vi "axex_save_file.vi"(7 "force operation (ignore error in) (True)":bool=TRUE, 8 "error in":errorcluster, 9 "file overwrite prompt (True)":bool=TRUE, 10 "file path (no path)":path, 11 "AX Excel instance in":T1) -> (0 "error out":errorcluster, 3 "AX Excel instance out":T1)   [LabVIEW 2020, in "AX Excel.lvlib"]
doc: "Call this to save unsaved changes in given file.\nIf current workbook is new workbook (not loaded from file) the file path must be entered.\nIf you want to change the save path from implicit (the path from which it was opened), you can enter new path."
uses:
  AX Excel.lvlib
  axex_instance.ctl
  <vilib>/Utility/error.llb/Error Cluster From Error Code.vi
  <vilib>/ErrorRing/Error Ring.xnode
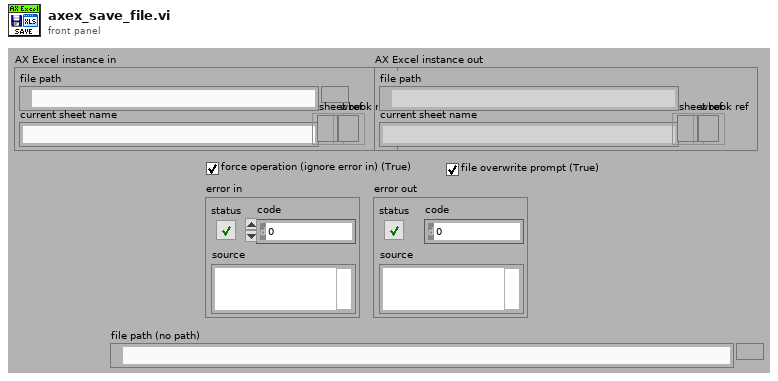
[diagram p1: front panel]
types:
  T1 = typedef "AX Excel.lvlib/axex_instance.ctl" = cluster{"file path":path, "current sheet name":string, "sheet ref":refnum<k7>, "wbook ref":refnum<k7>}
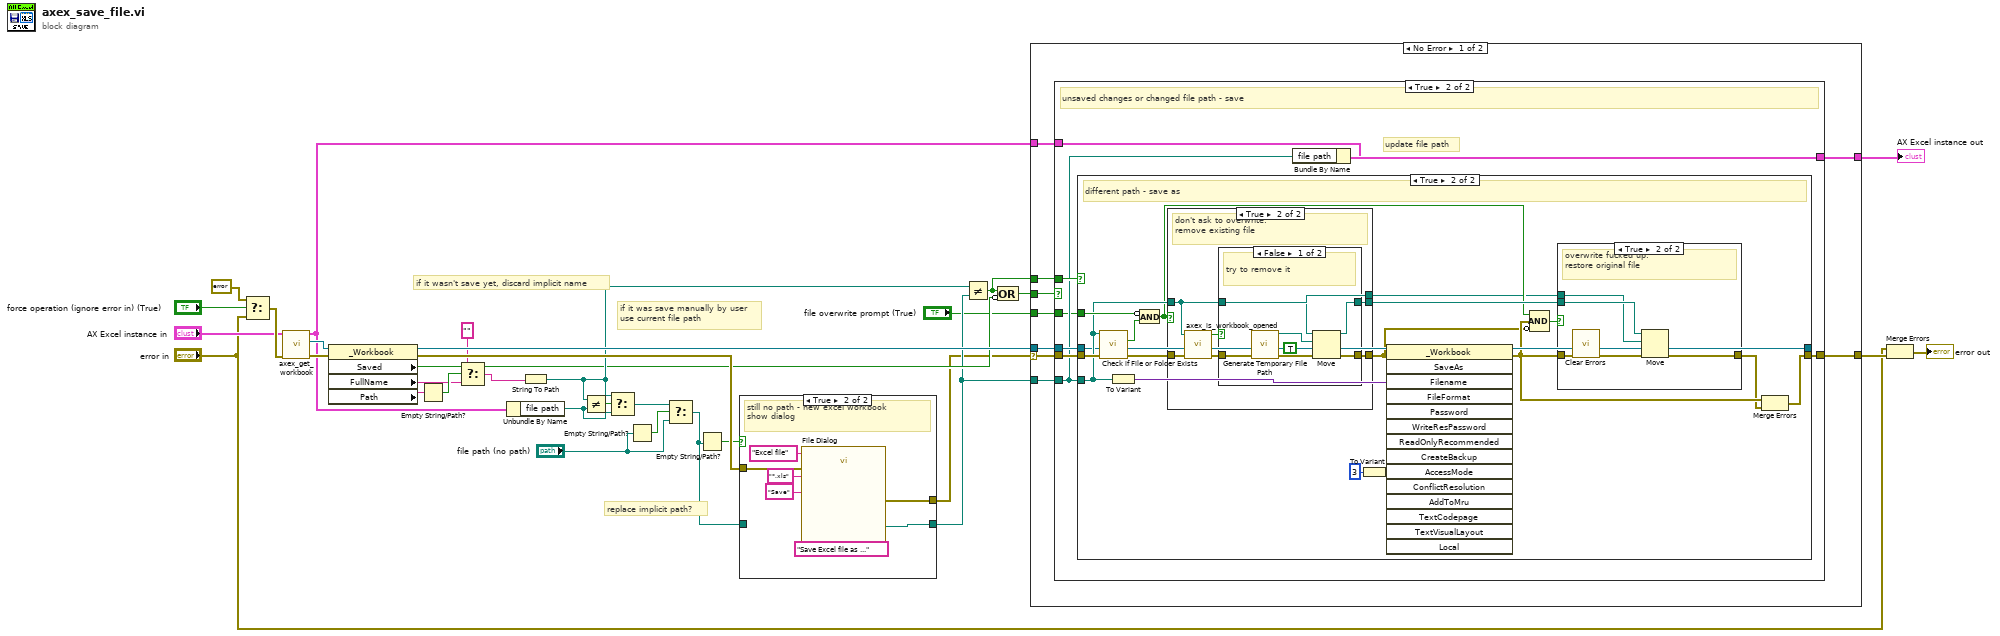
[diagram p0: block diagram]
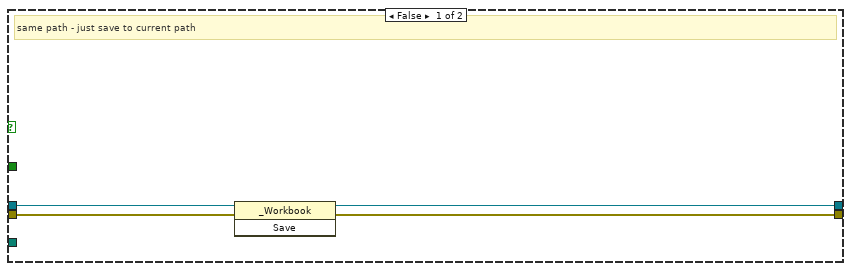
[diagram p3: hidden frame]
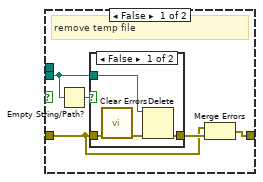
[diagram p4: hidden frame]
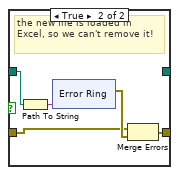
[diagram p7: hidden frame]
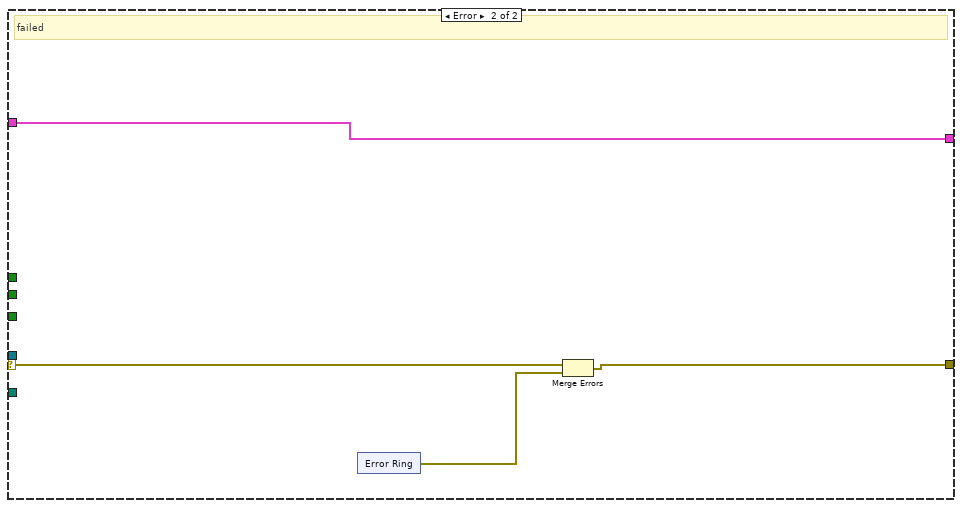
[diagram p8: hidden frame]
diagram:
  # "if it was save manually by user\nuse current file path"
  # "if it wasn't save yet, discard implicit name"
  # "replace implicit path?"
  n1 = Select(t=errorcluster {"status"=FALSE, "code"=0, "source"=""}, s="force operation (ignore error in) (True)", f="error in") -> (s? t:f=w30:errorcluster)
  n2 = call "axex_get_workbook.vi"("error in"=w30, "AX Excel instance in"="AX Excel instance in") -> ("error out"=w32:errorcluster, "excel workbook"=w25:refnum<k7>, "AX Excel instance out"=w8:T1)  [unwired: 7 in]
  n3 = property class="_Workbook"(reference=w25, error in=w32) -> (reference out=w31:refnum<k7>, error out=w19:errorcluster, "Saved"=w14:bool, "FullName"=w4:string, "Path"=w6:string)
  n4 = Empty String/Path?(string/path=w6) -> (empty?=w5:bool)
  n5 = Select(t="", s=w5, f=w4) -> (s? t:f=w2:string)
  n6 = Unbundle By Name(w8) -> ("file path"=w21:path)
  n7 = String To Path(string=w2) -> (path=w15:path)
  n8 = Not Equal?(x=w15, y=w21) -> (x != y?=w22:bool)
  n9 = Select(t=w15, s=w22, f=w21) -> (s? t:f=w20:path)
  n10 = Empty String/Path?(string/path="file path (no path)") -> (empty?=w24:bool)
  n11 = Select(t=w20, s=w24, f="file path (no path)") -> (s? t:f=w17:path)
  n12 = Empty String/Path?(string/path=w17) -> (empty?=w18:bool)
  n13 = case shown="True" w18 {
    tunnel: w19 -> [w34 w40]
    tunnel: [w34 w39] -> w11
    tunnel: [w33 w38] -> w12
    tunnel: w17 -> [w33 _]
    frame False {
      # "we have path - do nothing"
    }
    frame True {
      # "still no path - new excel workbook\nshow dialog"
      n14 = call "File Dialog"("prompt"="Save Excel file as ...", "button label"="Save", "error in"=w40, "pattern (all files)"="*.xls", "pattern label"="Excel file") -> ("selected path"=w38:path, "error out"=w39:errorcluster)  [unwired: 7 in, 2 out]
    }
  }
  n15 = Not Equal?(x=w15, y=w12) -> (x != y?=w13:bool)
  n16 = Compound Arithmetic op=OR(w13, invert w14) -> (w16:bool)
  n17 = case shown="No Error" w11 {
    selector: w11 -> [w46 w127]
    tunnel: w31 -> [w50 _]
    tunnel: w16 -> [w49 _]
    tunnel: w13 -> [w48 _]
    tunnel: w12 -> [w47 _]
    tunnel: [w45 w125] -> w10
    tunnel: [w44 w124] -> w9
    tunnel: w8 -> [w43 w124]
    tunnel: "file overwrite prompt (True)" -> [w42 _]
    frame No Error {
      n18 = case shown="True" w49 {
        tunnel: w50 -> [_ w60]
        tunnel: w46 -> [w52 w59]
        tunnel: w48 -> [_ w58]
        tunnel: w47 -> [_ w56]
        tunnel: [w52 w54] -> w45
        tunnel: [w51 w57] -> w44
        tunnel: w43 -> [w51 w55]
        tunnel: w42 -> [_ w53]
        frame False {
          # "no changes - no save"
        }
        frame True {
          # "update file path"
          # "unsaved changes or changed file path - save"
          n19 = case shown="True" w58 {
            tunnel: w59 -> [w64 w78]
            tunnel: w60 -> [w63 w73]
            tunnel: [w62 w67] -> w54
            tunnel: [w61 w82] -> _
            tunnel: w56 -> [_ w74]
            tunnel: w53 -> [_ w75]
            frame False {
              # "same path - just save to current path"
              n20 = invoke class="_Workbook" method="Save"(reference=w63, error in=w64) -> (reference out=w61:refnum<k7>, error out=w62:errorcluster)  [unwired: 1 in, 1 out]
            }
            frame True {
              # "different path - save as"
              n21 = call <vilib>:"Check if File or Folder Exists.vi"("error in (no error)"=w78, "path"=w74) -> ("error out"=w77:errorcluster, "file or folder exists?"=w76:bool)  [unwired: 7 in, 1 out]
              n22 = To Variant(anything=w74) -> (Variant=w81:variant)
              n23 = Compound Arithmetic op=AND(invert w75, w76) -> (w70:bool)
              n24 = case shown="True" w70 {
                tunnel: w77 -> [w98 w102]
                tunnel: [w98 w104] -> w65
                tunnel: w74 -> [_ w101]
                tunnel: [_ w103] -> w72
                tunnel: [_ w101] -> w66
                frame False {
                }
                frame True {
                  # "don't ask to overwrite:\nremove existing file"
                  n25 = call "axex_is_workbook_opened.vi"("error in"=w102, "path"=w101) -> ("error out"=w100:errorcluster, "is loaded?"=w99:bool)  [unwired: 8 in]
                  n26 = case shown="False" w99 {
                    tunnel: [w108 w116] -> w104
                    tunnel: [w107 _] -> w103
                    tunnel: w101 -> [w106 w112]
                    tunnel: w100 -> [w105 w114]
                    frame False {
                      # "try to remove it"
                      n27 = call <vilib>:"Generate Temporary File Path.vi"("error in (no error)"=w105) -> ("error out"=w111:errorcluster, "Unique Temporary File Path"=w110:path)  [unwired: 9 in]
                      n28 = Move(source path=w106, error in=w111, 9:TRUE ("overwrite (F)"), 10:w110) -> (error out=w108:errorcluster, 3:w107:path)  [unwired: 1 in, 1 out]
                    }
                    frame True {
                      # "the new file is loaded in Excel, so we can't remove it!"
                      n29 = Path To String(path=w112) -> (string=w113:string)
                      n30 = xnode "Error Ring"("parameter 0"=w113) -> ("error out"=w115:errorcluster)
                      n31 = Merge Errors(w114, w115) -> (w116:errorcluster)
                    }
                  }
                }
              }
              n32 = To Variant(anything=3) -> (Variant=w79:variant)
              n33 = invoke class="_Workbook" method="SaveAs"(reference=w73, error in=w65, "Filename"=w81, "ConflictResolution"=w79) -> (reference out=w82:refnum<k7>, error out=w69:errorcluster)  [unwired: 11 in, 13 out]
              n34 = Compound Arithmetic op=AND(w70, w69, invert w65) -> (w71:bool)
              n35 = case shown="True" w71 {
                tunnel: w69 -> [w84 w95]
                tunnel: [w83 w96] -> w68
                tunnel: w72 -> [w86 w97]
                tunnel: w66 -> [_ w93]
                frame False {
                  # "remove temp file"
                  n36 = Empty String/Path?(string/path=w86) -> (empty?=w87:bool)
                  n37 = case shown="False" w87 {
                    tunnel: w86 -> [w91 _]
                    tunnel: w84 -> [w90 w92]
                    tunnel: [w88 w92] -> w85
                    frame False {
                      n38 = call <vilib>:"Clear Errors.vi"("error in (no error)"=w90) -> ("error out"=w89:errorcluster)  [unwired: 5 in, 1 out]
                      n39 = Delete(path (use dialog)=w91, error in=w89) -> (error out=w88:errorcluster)  [unwired: 3 in, 2 out]
                    }
                    frame True {
                    }
                  }
                  n40 = Merge Errors(w84, w85) -> (w83:errorcluster)
                }
                frame True {
                  # "overwrite fucked up:\nrestore original file"
                  n41 = call <vilib>:"Clear Errors.vi"("error in (no error)"=w95) -> ("error out"=w94:errorcluster)  [unwired: 5 in, 1 out]
                  n42 = Move(source path=w97, error in=w94, 10:w93) -> (error out=w96:errorcluster)  [unwired: 2 in, 2 out]
                }
              }
              n43 = Merge Errors(w69, w68) -> (w67:errorcluster)
            }
          }
          n44 = Bundle By Name(cluster=w55, "file path"=w56) -> (w57:T1)
        }
      }
    }
    frame Error {
      # "failed"
      n45 = xnode "Error Ring"() -> ("error out"=w126:errorcluster)
      n46 = Merge Errors(w127, w126) -> (w125:errorcluster)
    }
  }
  "AX Excel instance out" <- w9
  n47 = Merge Errors("error in", w10) -> (→"error out":errorcluster)
